vi "LimelightDistance.vi"(10 "Moving Avg Size":i32=4) -> (2 "Distance (in)":dbl(slide)=18.87888327698158 scale=14.0..50.0)   [LabVIEW 2018]
doc: "This VI runs in parallel to other tasks. It can contain as many user-defined periodic loops as you need. These can carry out PID or other sorts of timed response."
uses:
  <vilib>/Rock Robotics/Network Tables/NT Read Numeric Array.vi
panel:
  in  "XY Tail":i32=10
  out "XY Graph":cluster{dbl[], dbl[]}(graph)={[1.5299748879521058, 1.5299748879521058, 1.5299748879521058, 1.5299748879521058, 1.5299748879521058, 1.5299748879521058, 1.5299748879521058, 1.5299748879521058, 1.5299748879521058, 1.5299748879521058], [-18.816785342563982, -18.816785342563982, -18.816785342563982, -18.816785342563982, -18.816785342563982, -18.816785342563982, -18.816785342563982, -18.816785342563982, -18.816785342563982, -18.816785342563982]}
  out "Z":cluster{"Numeric":dbl, dbl}(graph)={"Numeric"=-18.816785342563982, -18.816785342563982}
  out "X":cluster{"Numeric":dbl, dbl}(graph)={"Numeric"=1.5299748879521058, 1.5299748879521058}
  out "Avg Z":dbl=-18.816785342563982
  out "Avg X":dbl=1.5299748879521058
  out "Cam Tran Array":dbl[](array[numeric])=[1.5299748879521058, 3.615602048132313, -18.816785342563982, -6.502645805079064, 7.483339345520812, 4.672478071337118]
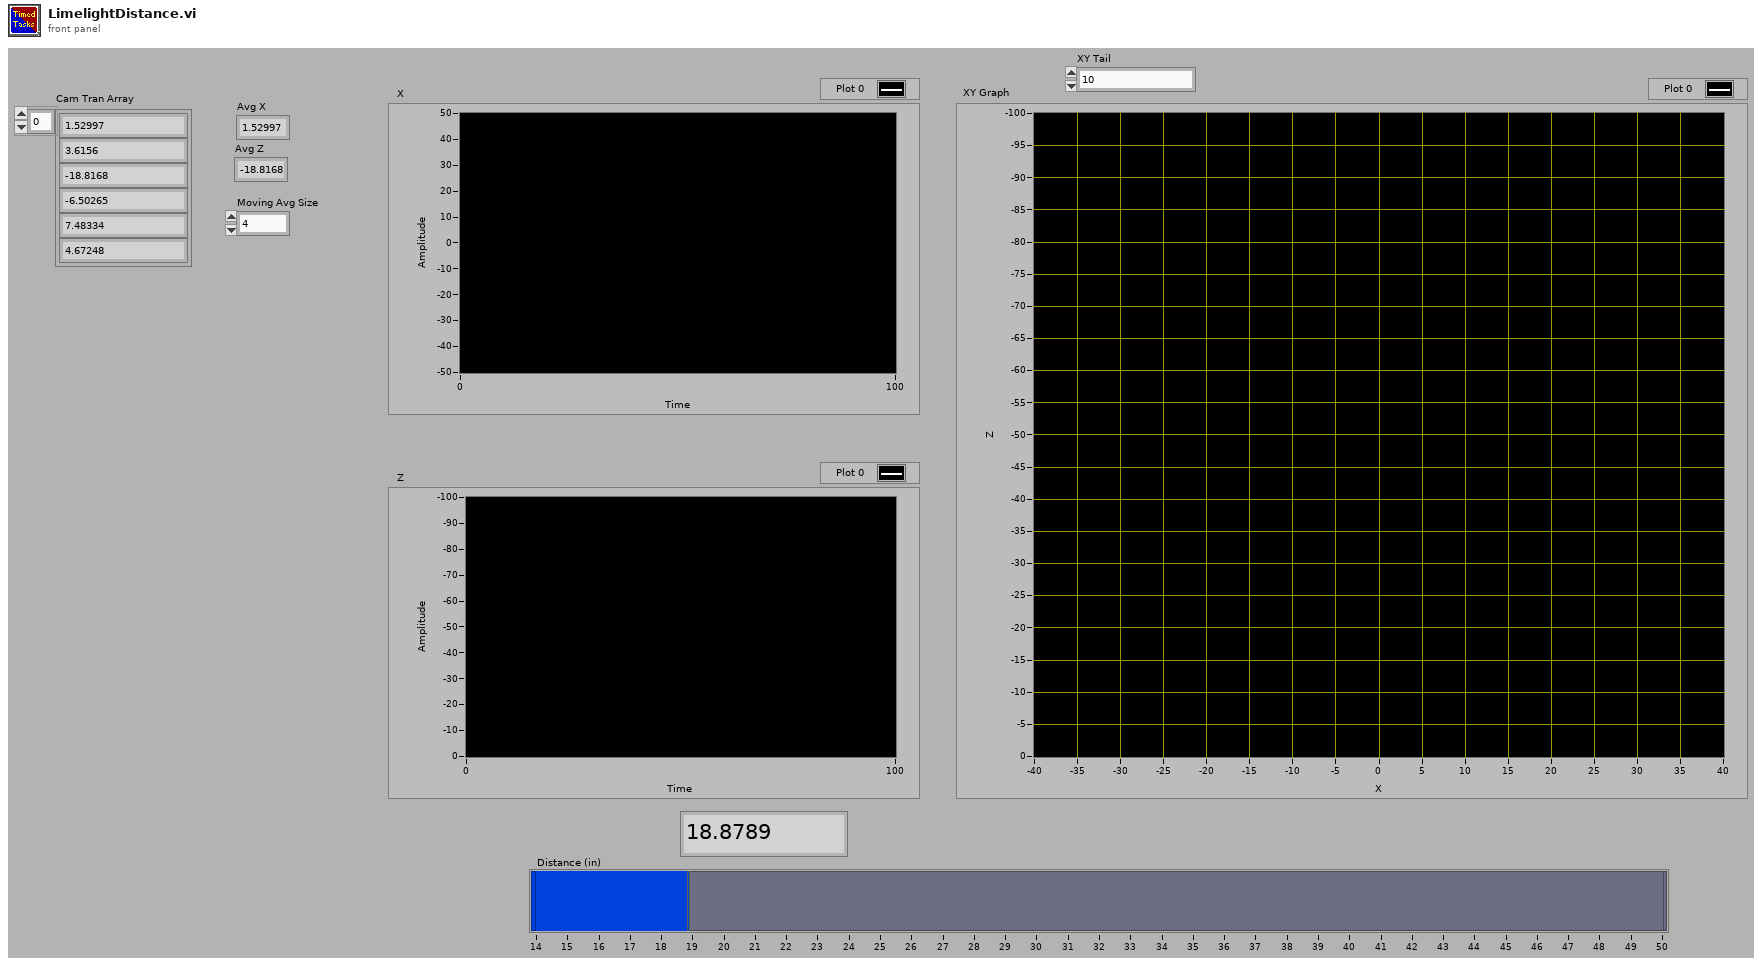
[diagram p1: front panel]
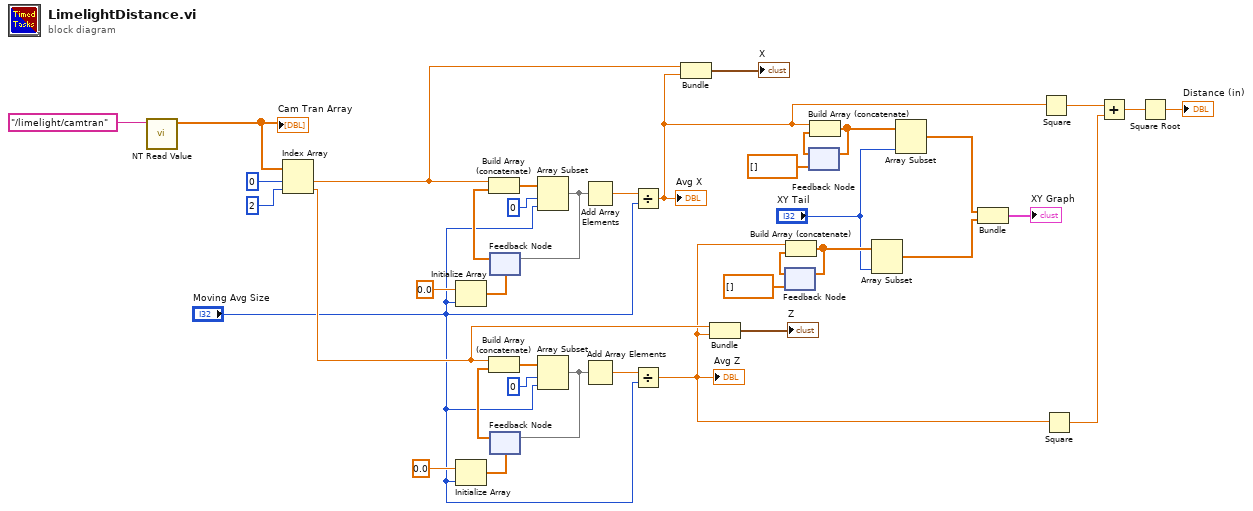
[diagram p0: block diagram]
diagram:
  n1 = call-poly <vilib>:"NT Read Value.vi"("Name"="/limelight/camtran") -> ("Numeric Array"=w38:dbl[])  [unwired: 9 in, 1 out]
  "Cam Tran Array" <- w38
  n2 = Index Array(array=w38, index #1=0 ("index"), index #2=2 ("index")) -> (element #1=w31:dbl, element #2=w19:dbl)
  n3 = Initialize Array(0.0 ("element"), "Moving Avg Size") -> (w34:dbl[])
  n4 = Initialize Array(0.0 ("element"), "Moving Avg Size") -> (w25:dbl[])
  n5 = feedback #1(w34) -> (w35:dbl[])
  n6 = Build Array (concatenate)(w31, w35) -> (w29:dbl[])
  n7 = feedback #2(w25) -> (w26:dbl[])
  n8 = Build Array (concatenate)(w19, w26) -> (w22:dbl[])
  n9 = Array Subset(array=w29, index=0, length="Moving Avg Size") -> (w27:dbl[])
  n10 = feedback-in #1(w27) -> ()
  n11 = Array Subset(array=w22, index=0, length="Moving Avg Size") -> (w20:dbl[])
  n12 = feedback-in #2(w20) -> ()
  n13 = Add Array Elements(numeric array=w27) -> (sum=w32:dbl)
  n14 = Add Array Elements(numeric array=w20) -> (sum=w23:dbl)
  n15 = Divide(x=w32, y="Moving Avg Size") -> (x/y=w6:dbl)
  "Avg X" <- w6
  n16 = Divide(x=w23, y="Moving Avg Size") -> (x/y=w5:dbl)
  "Avg Z" <- w5
  n17 = Bundle("Numeric"=w31, w6) -> (→"X":cluster{"Numeric":dbl, dbl})  [unwired: 1 in]
  n18 = Bundle("Numeric"=w19, w5) -> (→"Z":cluster{"Numeric":dbl, dbl})  [unwired: 1 in]
  n19 = feedback #3(dbl[] []) -> (w16:dbl[])
  n20 = Build Array (concatenate)(w5, w16) -> (w15:dbl[])
  n21 = feedback-in #3(w15) -> ()
  n22 = feedback #4(dbl[] []) -> (w13:dbl[])
  n23 = Build Array (concatenate)(w6, w13) -> (w12:dbl[])
  n24 = feedback-in #4(w12) -> ()
  n25 = Array Subset(array=w15, length="XY Tail") -> (w9:dbl[])  [unwired: 1 in]
  n26 = Array Subset(array=w12, length="XY Tail") -> (w8:dbl[])  [unwired: 1 in]
  n27 = Bundle(w8, w9) -> (→"XY Graph":cluster{dbl[], dbl[]})  [unwired: 1 in]
  n28 = Square(x=w6) -> (x^2=w4:dbl)
  n29 = Square(x=w5) -> (x^2=w3:dbl)
  n30 = Add(x=w4, y=w3) -> (x+y=w2:dbl)
  n31 = Square Root(x=w2) -> (sqrt(x)=→"Distance (in)":dbl)
